vi "3A PWM MotorControl.vi"() -> ()   [LabVIEW 2011]
uses:
  2-Think/2 Typedefs/rudder angle.ctl
  2-Think/2 Typedefs/sail setpt.ctl
  <vilib>/FPGAPlugInAG/cRIO-9113/niLvFpga_Open_cRIO-9113.vi
  2-Think/2 Globals/2 Global.vi
  <vilib>/Utility/error.llb/Error Cluster From Error Code.vi
  <vilib>/rvi/errors/niLvFpgaAdjustHostInterfaceError.vi
  <vilib>/FPGAPlugInAG/cRIO-9113/niLvFpga_Close_cRIO-9113.vi
  <vilib>/rvi/interface/nirviOpenFPGA/nirviOpenFPGA.xnode
  FPGA Bitfiles/SailBot_FPGATarget_3APWMMotorContro_81FD9E83.lvbitx
  FPGA/3A PWM MotorControl FPGA.vi
  <vilib>/rvi/interface/nirviReadWriteControl/nirviReadWriteControl.xnode
  <vilib>/rvi/interface/nirviCloseFPGA/nirviCloseFPGA.xnode
  FPGA Bitfiles/SailBot_FPGATarget3_3APWMMotorContro_1677D78E.lvbitx
  NiFpgaLv.dll
  <vilib>/FPGAPlugInAG/sbRIO-9606/niLvFpga_Open_sbRIO-9606.vi
panel:
  in  "Rudder Range":dbl=50.0
  in  "Rudder Trim":dbl(slide) scale=-20.0..20.0
  out "Sail Position":T1
  out "Rudder Angle":T2
  out "error out":errorcluster
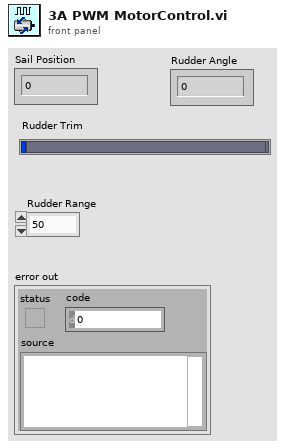
[diagram p1: front panel]
types:
  T1 = typedef "sail setpt.ctl" = dbl
  T2 = typedef "rudder angle.ctl" = dbl
  T3 = typedef "setpoints to boat.ctl" = cluster{"Sail Position":T1, "Rudder Angle":T2}
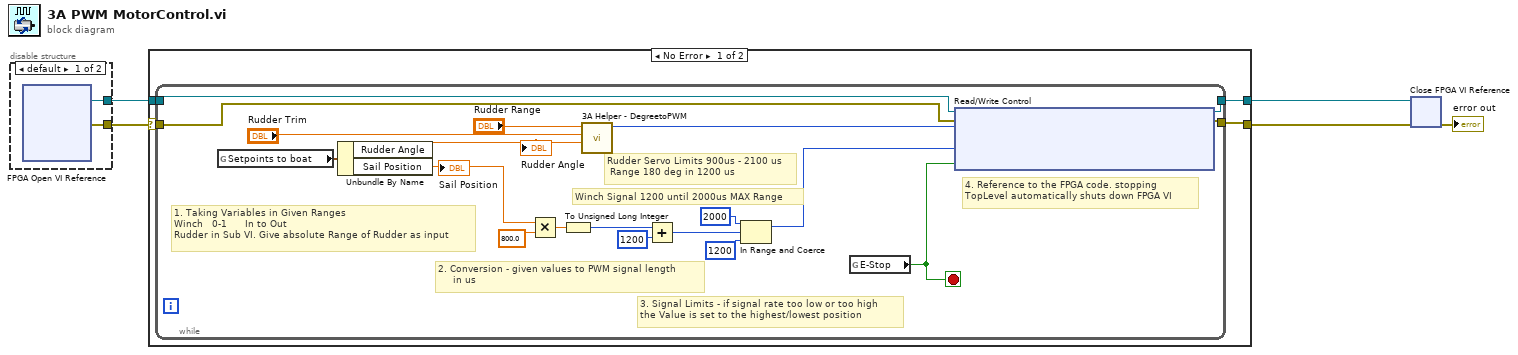
[diagram p0: block diagram]
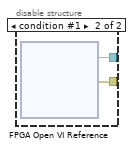
[diagram p2: hidden frame]
diagram:
  n1 = disable-structure shown="default" {
    disable-tunnel: [w6 w8] -> w4
    disable-tunnel: [w7 w9] -> w3
    frame condition #0 (active) {
      n2 = xnode "FPGA Open VI Reference"() -> ("FPGA VI Reference Out"=w6:refnum<k20>, "error out"=w7:errorcluster)  [unwired: 2 in]
    }
    frame condition #1 {
      n3 = xnode "FPGA Open VI Reference"() -> ("FPGA VI Reference Out"=w8:refnum<k20>, "error out"=w9:errorcluster)  [unwired: 2 in]
    }
  }
  n4 = case shown="No Error" w3 {
    selector: w3 -> [w13 w33]
    tunnel: [w10 w34] -> w2
    tunnel: [w11 w33] -> w1
    tunnel: w4 -> [w12 w34]
    frame No Error {
      n5 = while {
        tunnel: w12 -> [w28]
        tunnel: w13 -> [w29]
        tunnel: [w27] -> w11
        tunnel: [w26] -> w10
        stop <- w14 stop-if-true
        # "Rudder Servo Limits 900us - 2100 us\n Range 180 deg in 1200 us"
        # "1. Taking Variables in Given Ranges\nWinch   0-1      In to Out\nRudder in Sub VI. Give absolute Range of Rudder as input"
        # "2. Conversion - given values to PWM signal length\n     in us"
        # "3. Signal Limits - if signal rate too low or too high \nthe Value is set to the highest/lowest position"
        # "4. Reference to the FPGA code. stopping \nTopLevel automatically shuts down FPGA VI"
        # "Winch Signal 1200 until 2000us MAX Range"
        n6 = global read "2 Global.vi" "Setpoints to boat"() -> (w19:T3)
        n7 = Unbundle By Name(w19) -> ("Rudder Angle"=w18:T2, "Sail Position"=w16:T1)
        "Rudder Angle" <- w18
        "Sail Position" <- w16
        n8 = Multiply(x=w16, y=800.0) -> (x*y=w32:T1)
        n9 = To Unsigned Long Integer(number=w32) -> (unsigned 32bit integer=w31:u32)
        n10 = call "3A Helper - DegreetoPWM.vi"("Rudder Angle"=w18, "Rudder Trim"="Rudder Trim", "Rudder Range (deg)"="Rudder Range") -> ("Servo Position (us)"=w24:u32)  [unwired: 8 in]
        n11 = Add(x=w31, y=u32 1200) -> (x+y=w23:u32)
        n12 = In Range and Coerce(upper limit=u32 2000, x=w23, lower limit=u32 1200) -> (coerced(x)=w20:u32)  [unwired: 1 out]
        n13 = global read "2 Global.vi" "E-Stop"() -> (w14:bool)
        n14 = xnode "Read/Write Control"("FPGA VI Reference In"=w28, "error in"=w29, "SERVO 2 Duty in Ticks"=w24, "SERVO 1 Duty in Ticks"=w20, "stop PWM"=w14) -> ("FPGA VI Reference Out"=w26:refnum<k20>, "error out"=w27:errorcluster)
      }
    }
    frame Error {
      # "Error occurred. Do not run."
    }
  }
  n15 = xnode "Close FPGA VI Reference"("FPGA VI Reference In"=w2, "error in"=w1) -> ("error out"=→"error out":errorcluster)
